vi "Change to regular timebase.vi"(7 "NaN (unticked Interpolate)":bool, 8 "Sample Rate":i32, 9 "Data":dbl[][](array[numeric]) format="%.2f", 10 "Time":sgl[](array[numeric]) format="%.4f") -> (2 "Interp Data":dbl[][](array[numeric]) format="%.2f")   [LabVIEW 2016]
panel:
  in  "Max time":sgl
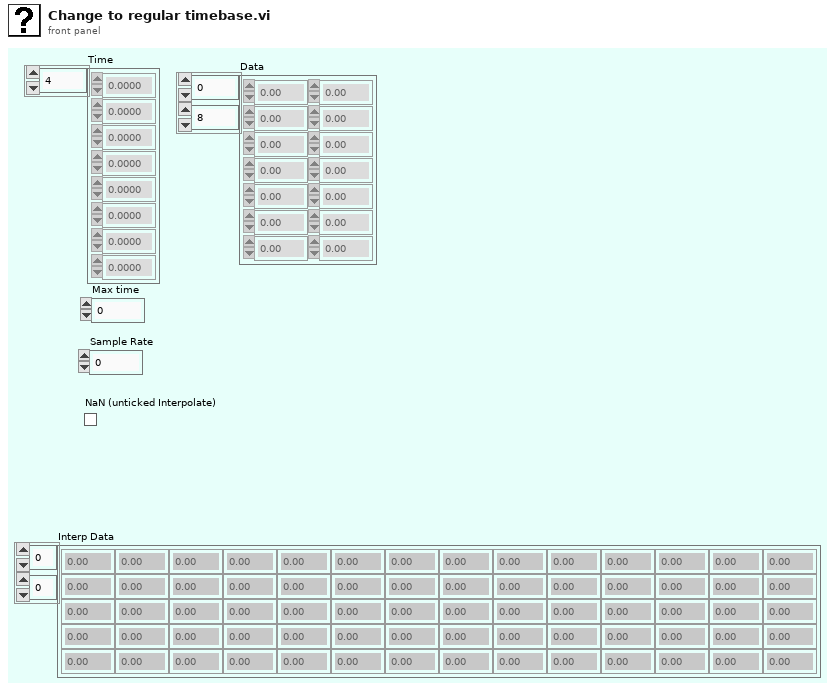
[diagram p1: front panel]
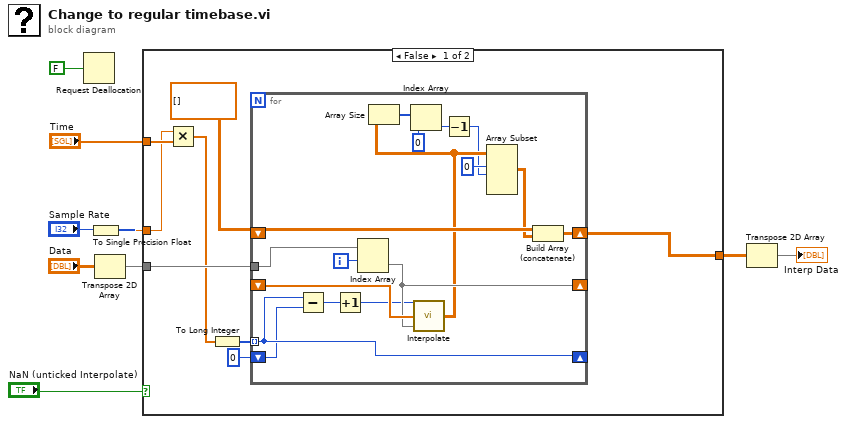
[diagram p0: block diagram]
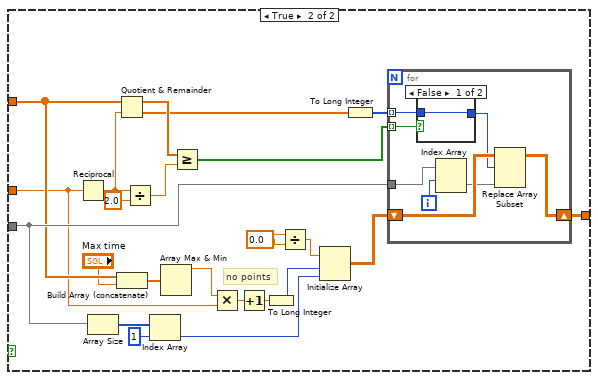
[diagram p2: hidden frame]
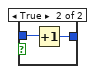
[diagram p3: hidden frame]
diagram:
  n1 = Request Deallocation(FALSE ("flag")) -> ()
  n2 = To Single Precision Float(number="Sample Rate") -> (single precision float=w4:sgl)
  n3 = Transpose 2D Array(2D array="Data") -> (transposed array=w2:dbl[][])
  n4 = case shown="False" "NaN (unticked Interpolate)" {
    tunnel: [w13 w54] -> w8
    tunnel: w2 -> [w16 w47]
    tunnel: "Time" -> [w11 w41]
    tunnel: w4 -> [w10 w36]
    frame False {
      n5 = Multiply(x=w10, y=w11) -> (x*y=w12:sgl[])
      n6 = To Long Integer(number=w12) -> (32bit integer=w14:i32[])
      n7 = for {
        tunnel: w14 -> [w34] mode=indexing
        shift-right: [w34] -> _
        shift-left: 0 -> [w33]
        shift-right: [w28] -> _
        shift-left: _ -> [w31]
        tunnel: w16 -> [w27]
        shift-right: [w30] -> w13
        shift-left: dbl[][] [] -> [w29]
        i -> [w18]
        n8 = Subtract(x=w34, y=w33) -> (x-y=w32:i32)
        n9 = Increment(x=w32) -> (x+1=w26:i32)
        n10 = Index Array(array=w27, index (row)=w18) -> (element=w28:dbl[])  [unwired: 1 in]
        n11 = call "Interpolate.vi"("Last Scan"=w28, "First Scan"=w31, "Length"=w26) -> ("Ramp Pattern"=w22:dbl[][])
        n12 = Array Size(array=w22) -> (size(s)=w25:i32[])
        n13 = Index Array(array=w25, index=0) -> (element=w23:i32)
        n14 = Decrement(x=w23) -> (x-1=w19:i32)
        n15 = Array Subset(array=w22, index (row)=0 ("index"), length (row)=w19) -> (w21:dbl[][])  [unwired: 2 in]
        n16 = Build Array (concatenate)(w29, w21) -> (w30:dbl[][])
      }
    }
    frame True {
      w56 = 0.0
      # "no points"
      n17 = Reciprocal(x=w36) -> (1/x=w44:sgl)
      n18 = Array Size(array=w47) -> (size(s)=w48:i32[])
      n19 = Quotient & Remainder(x=w41, y=w44) -> (x-y*floor(x/y)=w53:sgl[], floor(x/y)=w51:sgl[])
      n20 = Build Array (concatenate)(w41, "Max time") -> (w42:sgl[])
      n21 = Divide(x=w44, y=sgl 2.0) -> (x/y=w43:sgl)
      n22 = Index Array(array=w48, index=1) -> (element=w46:i32)
      n23 = Array Max & Min(array=w42) -> (max value=w37:sgl)  [unwired: 3 out]
      n24 = Greater Or Equal?(x=w53, y=w43) -> (x >= y?=w52:bool[])
      n25 = Multiply(x=w37, y=w36) -> (x*y=w39:sgl)
      n26 = Increment(x=w39) -> (x+1=w40:sgl)
      n27 = To Long Integer(number=w40) -> (32bit integer=w38:i32)
      n28 = Divide(x=w56, y=w56) -> (x/y=w57:dbl)
      n29 = Initialize Array(w57, w38, w46) -> (w55:dbl[][])
      n30 = To Long Integer(number=w51) -> (32bit integer=w50:i32[])
      n31 = for {
        tunnel: w47 -> [w61]
        shift-right: [w64] -> w54
        shift-left: w55 -> [w65]
        tunnel: w52 -> [w63] mode=indexing
        tunnel: w50 -> [w62] mode=indexing
        i -> [w58]
        n32 = case shown="False" w63 {
          tunnel: w62 -> [w66 w68]
          tunnel: [w66 w67] -> w59
          frame False {
          }
          frame True {
            n33 = Increment(x=w68) -> (x+1=w67:i32)
          }
        }
        n34 = Index Array(array=w61, index (row)=w58) -> (element=w60:dbl[])  [unwired: 1 in]
        n35 = Replace Array Subset(array=w65, new element=w60, index (row)=w59) -> (w64:dbl[][])  [unwired: 1 in]
      }
    }
  }
  n36 = Transpose 2D Array(2D array=w8) -> (transposed array=→"Interp Data":dbl[][])
